vi "Write Marker Colors.vi"(5 "Marker Colors":T1, 9 "Scale in":refnum<class "Scale.lvclass">) -> (3 "Scale out":refnum<class "Scale.lvclass">)   [LabVIEW 2014, in "Raspberry Pi Compatible Compiler for LabVIEW.lvlib" / "Scale.lvclass"]
uses:
  Scale.lvclass
  <vilib>/Utility/miscctls.llb/LVTextColorsTypeDef.ctl
  Scale.lvclass/Scale.ctl
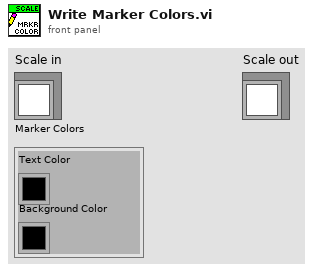
[diagram p1: front panel]
types:
  T1 = typedef "LVTextColorsTypeDef.ctl" = cluster{"Text Color":u32, "Background Color":u32}
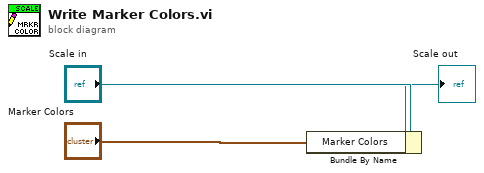
[diagram p0: block diagram]
diagram:
  n1 = Bundle By Name(cluster="Scale in", "Marker Colors"="Marker Colors") -> (→"Scale out":refnum<class "Scale.lvclass">)
